vi "myRIO_BRig_RT_dataCurrent_idxDataTrial.vi"() -> (2 "output_idxDataTrial":i32)   [LabVIEW 2014]
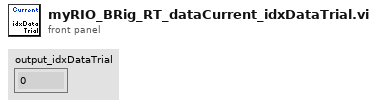
[diagram p1: front panel]
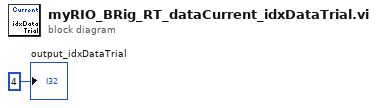
[diagram p0: block diagram]
diagram:
  "output_idxDataTrial" <- 4 ("output_iBlock")
